vi "set_request_query.vi"(8 "error in":errorcluster, 9 "value":string, 10 "key":string, 11 "obj in":refnum<class "RequestBuilder.lvclass">) -> (0 "error out":errorcluster, 2 "success":bool, 3 "obj out":refnum<class "RequestBuilder.lvclass">)   [LabVIEW 2020, in "reqwest.lvlib" / "RequestBuilder.lvclass"]
doc: "Use this to add search filters, pagination settings, or optional parameters to your API request URL (the ?page=1&limit=10 part) - it does NOT modify any headers and call it multiple times to build up all your query parameters."
uses:
  RequestBuilder.lvclass
  RequestBuilder.lvclass/RequestBuilder.ctl
  lv_reqwest_64.dll
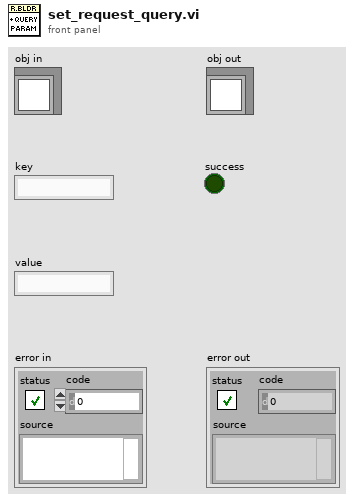
[diagram p1: front panel]
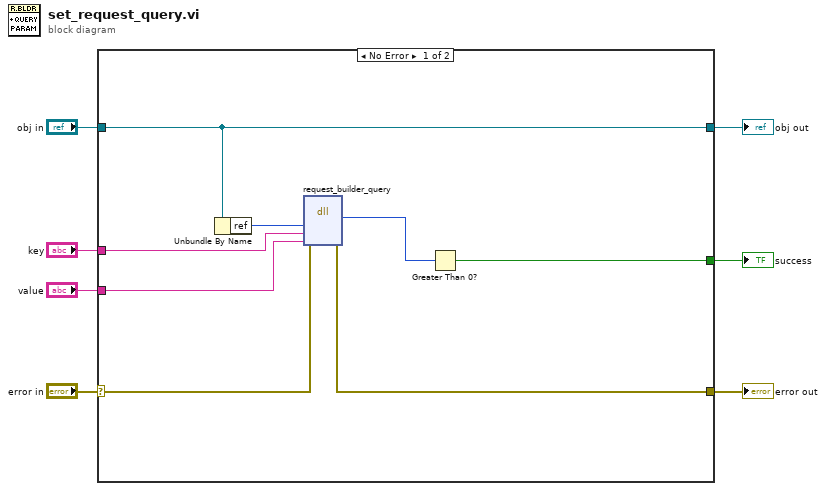
[diagram p0: block diagram]
diagram:
  n1 = case shown="No Error" "error in" {
    selector: "error in" -> [w15 w17]
    tunnel: "obj in" -> [w14 w16]
    tunnel: [w10 w17] -> w5
    tunnel: [w14 w16] -> w4
    tunnel: [w11 _] -> w3
    tunnel: "key" -> [w9 _]
    tunnel: "value" -> [w8 _]
    frame No Error {
      n2 = Unbundle By Name(w14) -> ("ref"=w13:u64)
      n3 = dll-call lib="C:/code/reqwest-rs-labview/lv_src/lv_reqwest_*.*" fn="request_builder_query"(error in=w15, "builder_ptr"=w13, "key"=w9, "value"=w8) -> (error out=w10:errorcluster, "Return Value"=w12:u8)  [unwired: 5 in, 1 out]
      n4 = Greater Than 0?(x=w12) -> (x > 0?=w11:bool)
    }
    frame Error {
    }
  }
  "error out" <- w5
  "obj out" <- w4
  "success" <- w3
